vi "Address Claim.vi"(8 "error in":errorcluster, 11 "J1939 Internals":T1={"J1939 XNET Settings"={"XNET Database"="", "XNET Cluster"="", "CAN port"="", "Baud rate [Bd]"=0, "J1939 Network Address"=0, "Name"=0, "Termination"=0}, "j1939 queues"={"Processed Outgoing"=refnum, "Process Outgoing"=refnum, "stop notifier"=refnum, "error queue"=refnum, "active dtc"=refnum, "processed inc"=refnum}, "fgv references"={"BAM Buffer"=refnum, "CM Buffer"=refnum, "CM Gen"=refnum, "BAM Gen"=refnum, "Address Claims"=refnum, "RQST"=refnum, "scaling lut"=refnum, "data lut"=refnum, "cyclic scheduler"=refnum}, "frame in"="", "frame out"="", "timing"={"tb to j1939 queue timeout"=100, "j1939 to tb queue timeout"=100, "dtc loop period (ms)"=100, "CAN in loop period (ms)"=100, "process incoming queue timeout (ms)"=100, "Outgoing Write Decimation"=0, "process outgoing loop rate (ms)"=0, "periodic outgoing queue timeout (ms)"=10, "CAN out queue timeout (ms)"=100}}) -> (0 "error out":errorcluster)   [LabVIEW 2013, in "J1939.lvlib"]
uses:
  J1939.lvlib
  API Types/Internal Data.ctl
  API Types/XNET Settings.ctl
  Users/Benjamin/Desktop/Tag bus J1939/J1939/RT Driver/J1939 Multi Packet Frame/_SubVIs/J1939 Setup Information Cluster.ctl
  API Types/CAN Outgoing Message Cluster.ctl
  Users/Benjamin/Desktop/Tag bus J1939/J1939/RT Driver/J1939 Multi Packet Frame/_SubVIs/J1939 Convert DTCs Cluster.ctl
  <vilib>/xnet/xnet.llb/XNET Frame CAN.ctl
  <vilib>/xnet/xnet.llb/XNET Frame Type CAN.ctl
  Users/Benjamin/Desktop/Tag bus J1939/J1939/RT Driver/J1939 Multi Packet Frame/_SubVIs/J1939 TP List References.ctl
  Users/Benjamin/Desktop/Tag bus J1939/J1939/RT Driver/J1939 Multi Packet Frame/_SubVIs/J1939 BAM Buffer Connections List_Ref.ctl
  Users/Benjamin/Desktop/Tag bus J1939/J1939/RT Driver/J1939 Multi Packet Frame/_SubVIs/J1939 Connection Mode Generation Connection Ref.ctl
  Users/Benjamin/Desktop/Tag bus J1939/J1939/RT Driver/J1939 Multi Packet Frame/_SubVIs/J1939 BAM Generation Connections List_Ref.ctl
  LUTs/J1939 Address Table Reference.ctl
  Users/Benjamin/Desktop/Tag bus J1939/J1939/RT Driver/J1939 Multi Packet Frame/_SubVIs/J1939 RQST Lookup Table Reference.ctl
  LUTs/J1939 Conversion Lookup Table Reference.ctl
  LUTs/J1939 Data Lookup Table Reference.ctl
  LUTs/Cyclic Frame Scheduler Lut Reference.ctl
  Configuration/TypeDefs/timing configuration.ctl
  LUTs/J1939 Address Lookup Table Action.ctl
  Frame Conversion/Convert CAN Data (U8) to U32.vi
  Frame Conversion/Convert CAN Data (U32) to U8.vi
  Frame Conversion/Convert CAN Arb ID to J1939 ID.vi
  Frame Conversion/Convert J1939 ID to CAN Arb ID.vi
  <vilib>/xnet/xnet.llb/XNET Write (Frame CAN).vi
  Common Messages/J1939 Message Request Address.vi
  <vilib>/xnet/xnet.llb/XNET Read.vi
  <vilib>/xnet/xnet.llb/XNET Read (Frame CAN).vi
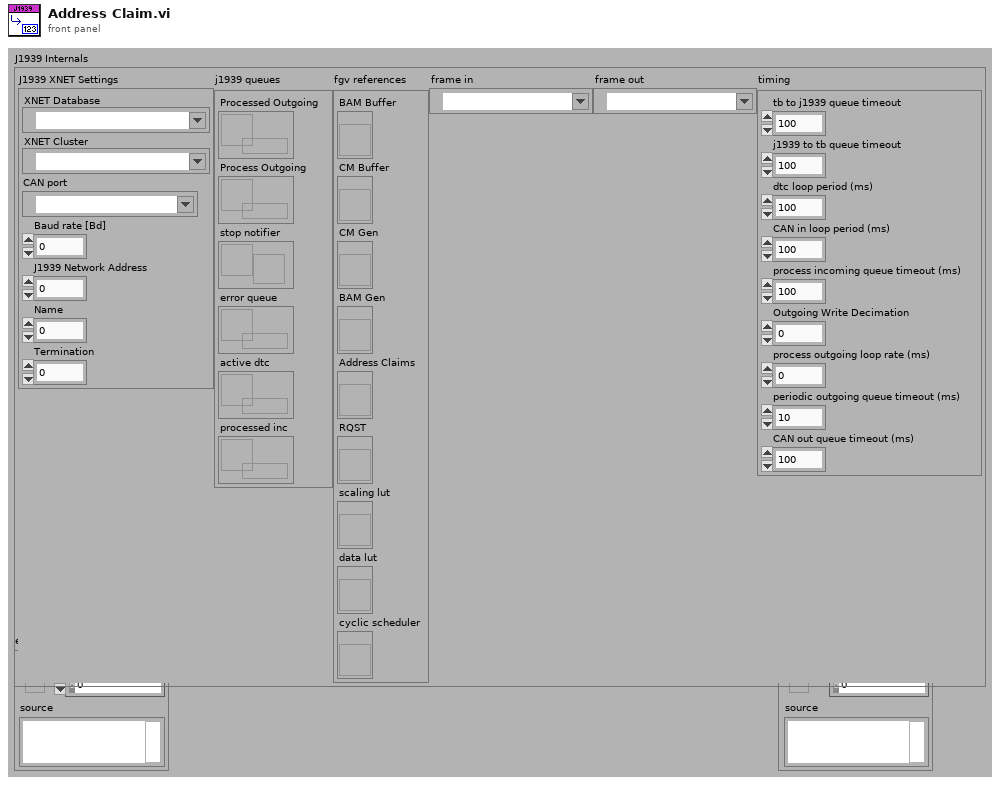
[diagram p1: front panel]
types:
  T1 = typedef "J1939.lvlib/Internal Data.ctl" = cluster{"J1939 XNET Settings":T2, "j1939 queues":T3, "fgv references":T4, "frame in":refnum<k21>, "frame out":refnum<k21>, "timing":T13}
  T2 = typedef "J1939.lvlib/XNET settings.ctl" = cluster{"XNET Database":refnum<k21>, "XNET Cluster":refnum<k21>, "CAN port":refnum<k21>, "Baud rate [Bd]":u32, "J1939 Network Address":u8, "Name":u64, "Termination":u32}
  T3 = typedef "J1939.lvlib/J1939 Setup Information Cluster.ctl" = cluster{"Processed Outgoing":refnum<queue>, "Process Outgoing":refnum<queue>, "stop notifier":refnum<notifier>, "error queue":refnum<queue>, "active dtc":refnum<queue>, "processed inc":refnum<queue>}
  T4 = typedef "J1939.lvlib/J1939 TP List References.ctl" = cluster{"BAM Buffer":T5, "CM Buffer":T5, "CM Gen":T6, "BAM Gen":T7, "Address Claims":T8, "RQST":T9, "scaling lut":T10, "data lut":T11, "cyclic scheduler":T12}
  T5 = typedef "J1939.lvlib/J1939 BAM Buffer Connections List_Ref.ctl" = refnum<vi>
  T6 = typedef "J1939.lvlib/J1939 Connection Mode Generation Connection Ref.ctl" = refnum<vi>
  T7 = typedef "J1939.lvlib/J1939 BAM Generation Connections List_Ref.ctl" = refnum<vi>
  T8 = typedef "J1939.lvlib/J1939 Address Table Reference.ctl" = refnum<vi>
  T9 = typedef "J1939.lvlib/J1939 RQST Lookup Table Reference.ctl" = refnum<vi>
  T10 = typedef "J1939.lvlib/J1939 Conversion Lookup Table Reference.ctl" = refnum<vi>
  T11 = typedef "J1939.lvlib/J1939 Data Lookup Table Reference.ctl" = refnum<vi>
  T12 = typedef "J1939.lvlib/cyclic frame scheduler lut reference.ctl" = refnum<vi>
  T13 = typedef "J1939.lvlib/timing configuration.ctl" = cluster{"tb to j1939 queue timeout":i32, "j1939 to tb queue timeout":i32, "dtc loop period (ms)":i32, "CAN in loop period (ms)":i32, "process incoming queue timeout (ms)":i32, "Outgoing Write Decimation":u32, "process outgoing loop rate (ms)":i32, "periodic outgoing queue timeout (ms)":i32, "CAN out queue timeout (ms)":i32}
  T14 = typedef "J1939.lvlib/CAN Outgoing Message Cluster.ctl" = cluster{"Identifier":u32, "Data":u8[]}
  T15 = typedef "XNET Frame CAN.ctl" = cluster{"timestamp":timestamp, "payload":u8[], "identifier":u32, "type":T16, "extended?":bool, "echo?":bool}
  T16 = typedef "XNET Frame Type CAN.ctl" = u8
  T17 = typedef "J1939.lvlib/Convert CAN Data (U8) Cluster.ctl" = cluster{"Byte 1":u8, "Byte 2":u8, "Byte 3":u8, "Byte 4":u8, "Byte 5":u8, "Byte 6":u8, "Byte 7":u8, "Byte 8":u8}
  T18 = typedef "J1939.lvlib/J1939 Address Lookup Table Action.ctl" = enum16{"Initialize", "Add", "Get", "Remove", "Get All"}
  T19 = typedef "J1939.lvlib/J1939 Address Lookup Table Data.ctl" = cluster{"Name":u8[], "Address":u8}
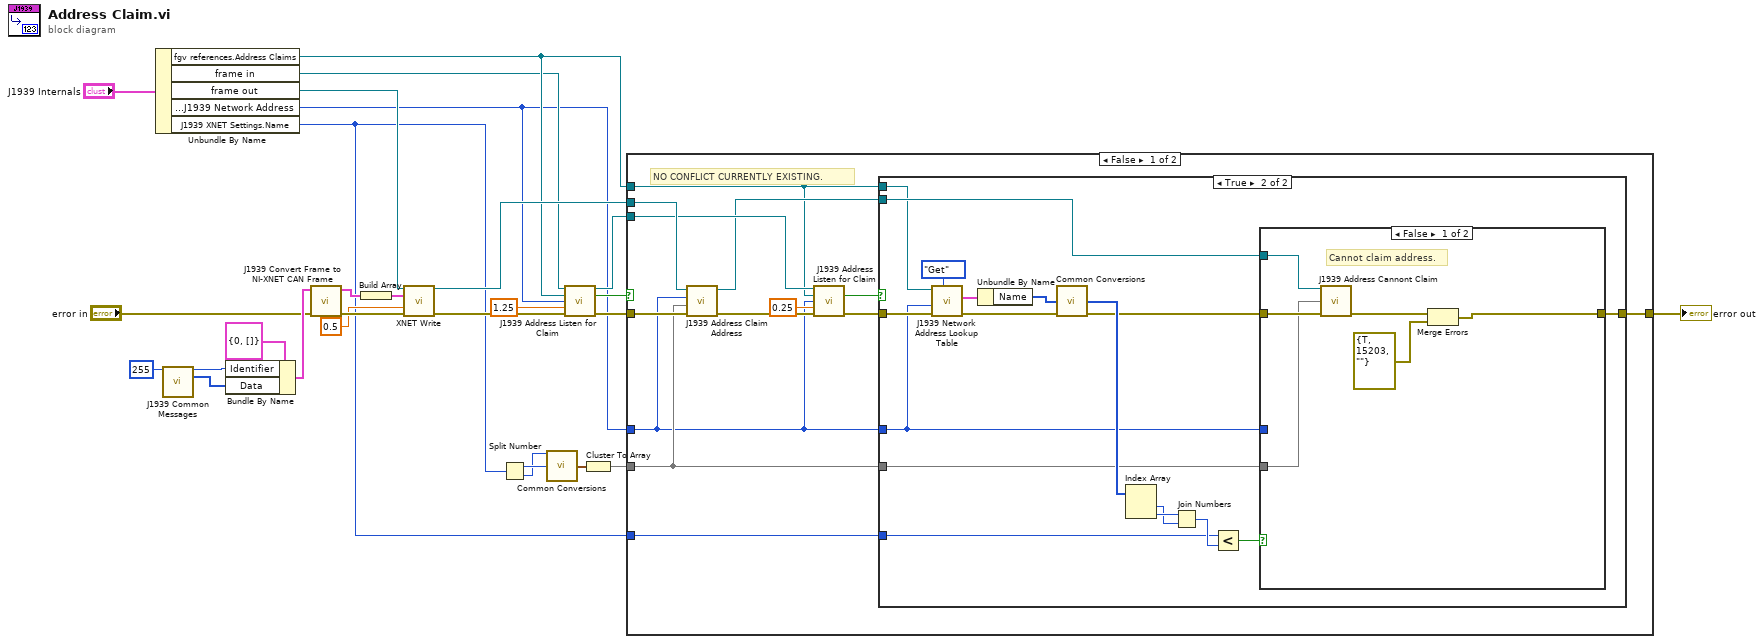
[diagram p0: block diagram]
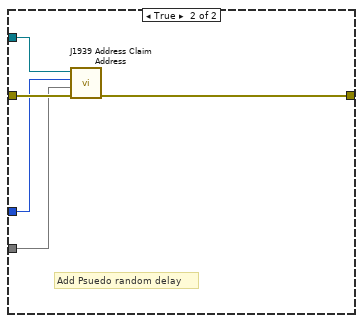
[diagram p3: hidden frame]
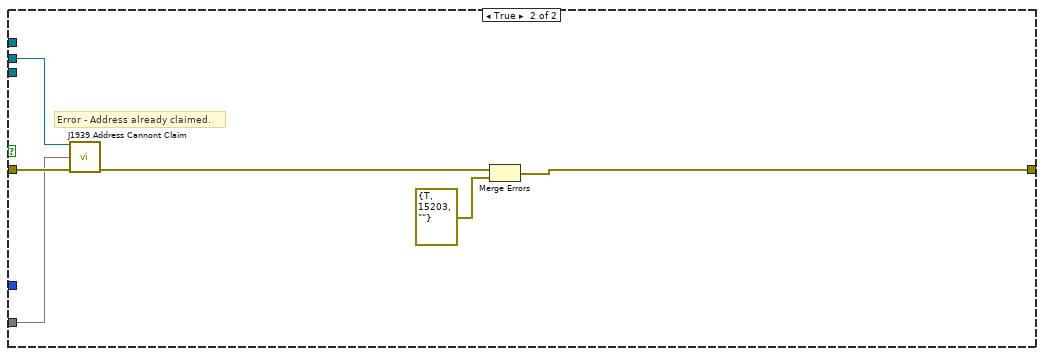
[diagram p4: hidden frame]
diagram:
  n1 = Unbundle By Name("J1939 Internals") -> ("fgv references.Address Claims"=w5:T8, "frame in"=w4:refnum<k21>, "frame out"=w3:refnum<k21>, "J1939 XNET Settings.J1939 Network Address"=w1:u8, "J1939 XNET Settings.Name"=w2:u64)
  n2 = call-poly "J1939 Common Messages.vi"("Destination Address"=u8 255) -> ("Arb ID"=w27:u32, "Data"=w26:u8[])  [unwired: 13 in]
  n3 = Bundle By Name(cluster=T14 {"Identifier"=0, "Data"=[]} ("Data to Send"), "Identifier"=w27, "Data"=w26) -> (w24:T14)
  n4 = call "J1939 Convert Frame to NI-XNET CAN Frame.vi"("error in"="error in", "Data to Send"=w24) -> ("error out"=w22:errorcluster, "CAN frame"=w23:T15)  [unwired: 8 in]
  n5 = Build Array(w23) -> (w9:T15[])
  n6 = call-poly <vilib>:"XNET Write.vi"("session in"=w3, "data"=w9, "timeout (10)"=0.5, "error in (no error)"=w22) -> ("session out"=w16:refnum<k21>, "error out"=w21:errorcluster)  [unwired: 10 out]
  n7 = Split Number(x=w2) -> (hi(x)=w14:u32, lo(x)=w13:u32)
  n8 = call-poly "Common Conversions.vi"("Data 0-3"=w13, "Data 4-7"=w14) -> ("Byte Cluster"=w15:T17)  [unwired: 13 in]
  n9 = call "J1939 Address Listen for Claim.vi"("session in"=w4, "ref in"=w5, "Requested Address"=w1, "timeout (0)"=1.25, "error in"=w21) -> ("session out"=w18:refnum<k21>, "Conflict?"=w19:bool, "error out"=w17:errorcluster)  [unwired: 8 in]
  n10 = Cluster To Array(cluster=w15) -> (array=w12:u8[])
  n11 = case shown="False" w19 {
    tunnel: w1 -> [w28 _]
    tunnel: w2 -> [w35 _]
    tunnel: w18 -> [w37 _]
    tunnel: w17 -> [w38 w74]
    tunnel: w16 -> [w39 w72]
    tunnel: [w31 w69] -> w7
    tunnel: w12 -> [w30 w73]
    tunnel: w5 -> [w29 _]
    frame False {
      # "NO CONFLICT CURRENTLY EXISTING."
      n12 = call "J1939 Address Claim Address.vi"("error in"=w38, "Byte Cluster"=w30, "Requested Address"=w28, "Write Session"=w39) -> ("error out"=w40:errorcluster, "Write Session out"=w33:refnum<k21>)  [unwired: 6 in]
      n13 = call "J1939 Address Listen for Claim.vi"("session in"=w37, "ref in"=w29, "Requested Address"=w28, "timeout (0)"=0.25, "error in"=w40) -> ("Conflict?"=w34:bool, "error out"=w32:errorcluster)  [unwired: 8 in, 1 out]
      n14 = case shown="True" w34 {
        tunnel: w35 -> [_ w45]
        tunnel: w33 -> [_ w53]
        tunnel: w32 -> [w41 w48]
        tunnel: w30 -> [_ w51]
        tunnel: [w41 w50] -> w31
        tunnel: w29 -> [_ w46]
        tunnel: w28 -> [_ w42]
        frame False {
          # "We have a valid address."
        }
        frame True {
          n15 = call "J1939 Network Address Lookup Table.vi"("Action"=J1939_Address_Lookup_Table_Action."Get", "error in (no error)"=w48, "Address"=w42, "ref in"=w46) -> ("error out"=w47:errorcluster, "Data"=w44:T19)  [unwired: 4 in, 2 out]
          n16 = Unbundle By Name(w44) -> ("Name"=w43:u8[])
          n17 = call-poly "Common Conversions.vi"("Data"=w43) -> ("Array"=w57:u32[])  [unwired: 14 in]
          n18 = Index Array(array=w57) -> (element #1=w55:u32, element #2=w56:u32)  [unwired: 2 in]
          n19 = Join Numbers(hi=w56, lo=w55) -> ((hi.lo)=w54:u64)
          n20 = Less?(x=w45, y=w54) -> (x < y?=w52:bool)
          n21 = case shown="False" w52 {
            tunnel: w53 -> [w61 w67]
            tunnel: w47 -> [w63 w68]
            tunnel: w51 -> [w62 w65]
            tunnel: [w58 w64] -> w50
            tunnel: w42 -> [_ w66]
            frame False {
              # "Cannot claim address."
              n22 = call "J1939 Address Cannont Claim.vi"("session out"=w61, "Byte Cluster"=w62, "error in"=w63) -> ("error out"=w60:errorcluster)  [unwired: 12 in]
              n23 = Merge Errors(w60, errorcluster {"status"=TRUE, "code"=15203, "source"=""} ("error out")) -> (w58:errorcluster)
            }
            frame True {
              # "Add Psuedo random delay"
              n24 = call "J1939 Address Claim Address.vi"("error in"=w68, "Byte Cluster"=w65, "Requested Address"=w66, "Write Session"=w67) -> ("error out"=w64:errorcluster)  [unwired: 6 in, 1 out]
            }
          }
        }
      }
    }
    frame True {
      # "Error - Address already claimed."
      n25 = call "J1939 Address Cannont Claim.vi"("session out"=w72, "Byte Cluster"=w73, "error in"=w74) -> ("error out"=w70:errorcluster)  [unwired: 12 in]
      n26 = Merge Errors(w70, errorcluster {"status"=TRUE, "code"=15203, "source"=""} ("error out")) -> (w69:errorcluster)
    }
  }
  "error out" <- w7
